vi "Loop.vi"(9 "Error Queue":refnum<queue>, 10 "Event Actor Queue":refnum<queue>, 11 "Event Actor in":refnum<class "Event Actor.lvclass">) -> ()   [LabVIEW 2021, in "Event Actor.lvclass"]
uses:
  Event Actor.lvclass
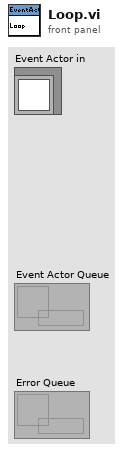
[diagram p1: front panel]
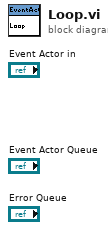
[diagram p0: block diagram]
diagram:
